vi "P4CMD NoOp.vi"(8 "error in (no error)":errorcluster) -> (0 "error out":errorcluster)   [LabVIEW 2017, in "NI_SCC_P4CMD.lvlib"]
uses:
  <vilib>/SourceControl/Providers/P4CMD/NI_SCC_P4CMD.lvlib
  <vilib>/SourceControl/Providers/P4CMD/P4CMD Close Project.vi
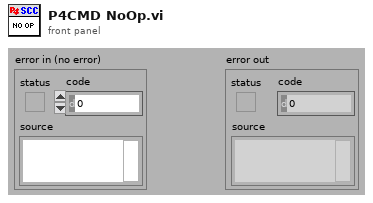
[diagram p1: front panel]
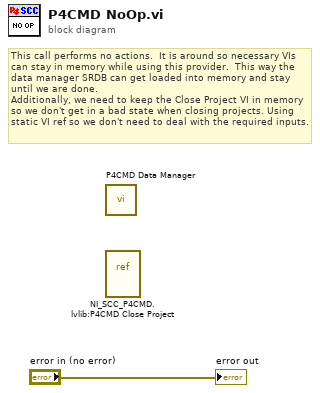
[diagram p0: block diagram]
diagram:
  # "This call performs no actions.  It is around so necessary VIs can stay in memory while using this provider.  This way the data manager SRDB can get loaded into memory and stay until we are done. \nAdditionally, we need to keep the Close Project VI in memory so we don't get in a bad state when closing projects. Using static VI ref so we don't need to deal with the required inputs."
  n1 = call <vilib>:"P4CMD Data Manager.vi"() -> ()  [unwired: 6 in, 6 out]
  n2 = vi-ref "NI_SCC_P4CMD.lvlib:P4CMD Close Project.vi"() -> ()  [unwired: 1 out]
  "error out" <- "error in (no error)"
